vi "Get User Interface VI.vi"(8 "error in (no error)":errorcluster, 11 "UDP Transfer Tx User Interface in":refnum<class "UDP Transfer Tx User Interface.lvclass">) -> (0 "error out":errorcluster, 2 "user interface vi":refnum<vi>, 3 "UDP Transfer Tx User Interface out":refnum<class "UDP Transfer Tx User Interface.lvclass">)   [LabVIEW 2017, in "UDP Transceiver.lvlib" / "UDP Transfer Tx User Interface.lvclass"]
uses:
  UDP Transfer Tx User Interface.lvclass
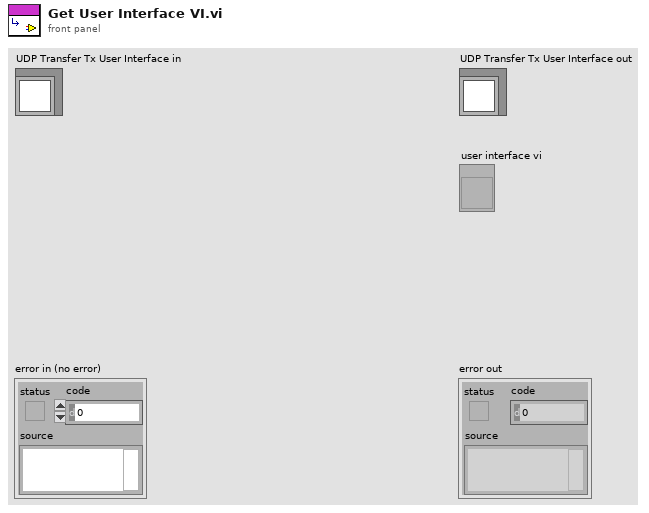
[diagram p1: front panel]
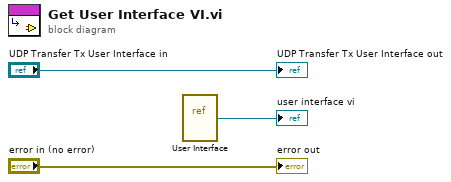
[diagram p0: block diagram]
diagram:
  n1 = vi-ref "User Interface.vi"() -> (→"user interface vi":refnum<vi>)
  "error out" <- "error in (no error)"
  "UDP Transfer Tx User Interface out" <- "UDP Transfer Tx User Interface in"
